vi "DC_CNTRL_select_module.vi"(7 "Read Answer?":bool, 8 "error in (no error)":errorcluster, 10 "Module number":i32, 11 "Handle":u64) -> (0 "error out":errorcluster, 3 "Handle out":u64)   [LabVIEW 2019]
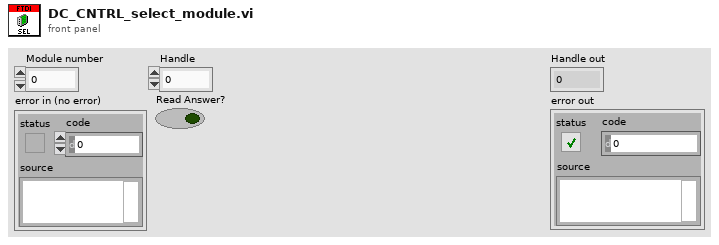
[diagram p1: front panel]
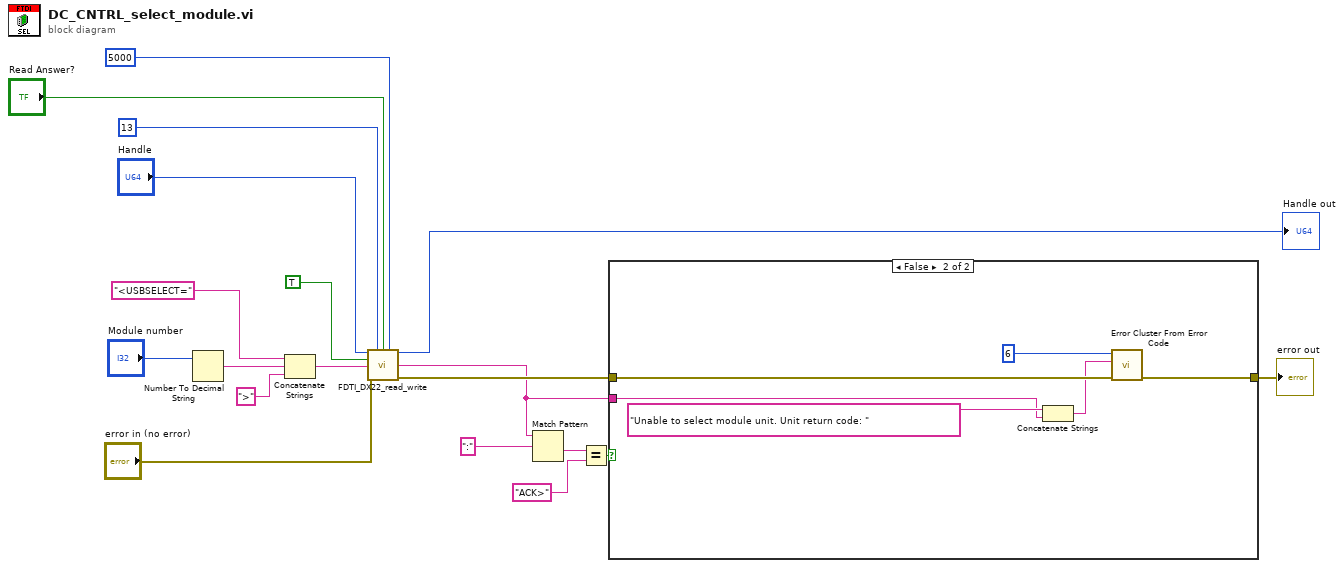
[diagram p0: block diagram]
diagram:
  n1 = Number To Decimal String(number="Module number") -> (decimal integer string=w17:string)  [unwired: 1 in]
  n2 = Concatenate Strings("<USBSELECT=" ("string"), w17, ">" ("string")) -> (w19:string)
  n3 = call "FDTI_DX22_read_write.vi"("Handle"="Handle", "Bytes to wait for"=13, "Read Answer?"="Read Answer?", "Bytes wait timeout / ms"=5000, "Clear  RxTx Buffer?"=TRUE, "Write string"=w19, "error in (no error)"="error in (no error)") -> ("Handle out"=→"Handle out":u64, "Read Data"=w2:string, "error out"=w7:errorcluster)  [unwired: 6 in]
  n4 = Match Pattern(string=w2, regular expression=":") -> (after substring=w5:string)  [unwired: 1 in, 3 out]
  n5 = Equal?(x=w5, y="ACK>") -> (x = y?=w4:bool)
  n6 = case shown="False" w4 {
    tunnel: w7 -> [w20 w26]
    tunnel: w2 -> [_ w24]
    tunnel: [w20 w21] -> w1
    frame True {
    }
    frame False {
      n7 = Concatenate Strings("Unable to select module unit. Unit return code: " ("string"), w24) -> (w23:string)
      n8 = call <vilib>:"Error Cluster From Error Code.vi"("error in (no error)"=w26, "error message (\"\")"=w23, "error code (0)"=6) -> ("error out"=w21:errorcluster)  [unwired: 6 in]
    }
  }
  "error out" <- w1
